vi "Stop all movement.vi"(8 "error in (no error)":errorcluster, 11 "Scientifica XYZ Gen1 in":refnum<class "Scientifica XYZ Gen1.lvclass">) -> (0 "error out":errorcluster, 2 "XYZ Position Set":T1={"Speed"=0, "Z Limit (um+/-)"=0.0, "Axes"="All", "XYZ Coordinates"={"X"=0.0, "Y"=0.0, "Z"=0.0}} {"XYZ Coordinates"."Z" format="Z= %#_g"; "XYZ Coordinates"."Y" format="Y= %#_g"; "XYZ Coordinates"."X" format="X= %#_g"; "Z Limit (um+/-)" format="Z Limit = %.0f"; "Speed" format="Speed= %.0f"}, 3 "Scientifica XYZ Gen1 out":refnum<class "Scientifica XYZ Gen1.lvclass">)   [LabVIEW 2020, in "TranslationStageClassStructure.lvlib" / "Scientifica XYZ Gen1.lvclass"]
uses:
  Scientifica XYZ Gen1.lvclass
  XYZ Stage Control/typedefs/XYZ_position_input.ctl
  XYZ Stage Control/typedefs/XYZ axes.ctl
  Typedefs/XYZ_coordinates.ctl
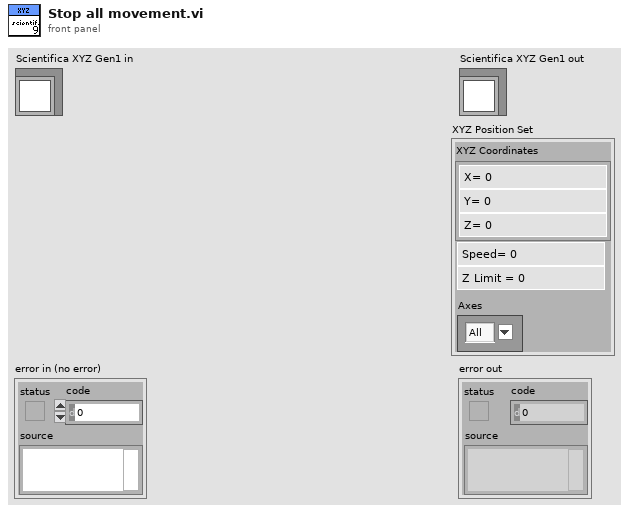
[diagram p1: front panel]
types:
  T1 = typedef "XYZ_position_input.ctl" = cluster{"Speed":i32, "Z Limit (um+/-)":sgl, "Axes":T2, "XYZ Coordinates":T3}
  T2 = typedef "XYZ axes.ctl" = string
  T3 = typedef "XYZ_coordinates.ctl" = cluster{"X":sgl, "Y":sgl, "Z":sgl}
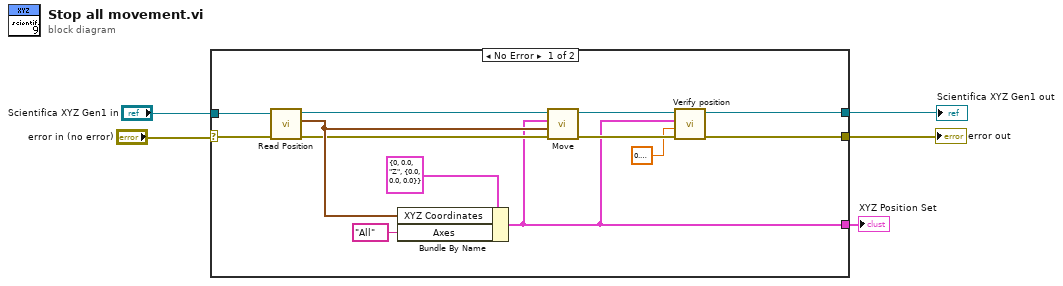
[diagram p0: block diagram]
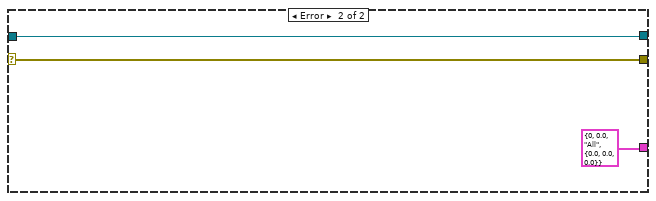
[diagram p2: hidden frame]
diagram:
  n1 = case shown="No Error" "error in (no error)" {
    selector: "error in (no error)" -> [w17 w21]
    tunnel: [w7 w21] -> w4
    tunnel: "Scientifica XYZ Gen1 in" -> [w18 w20]
    tunnel: [w9 w20] -> w2
    tunnel: [w6 T1 {"Speed"=0, "Z Limit (um+/-)"=0.0, "Axes"="All", "XYZ Coordinates"={"X"=0.0, "Y"=0.0, "Z"=0.0}} ("XYZ Position Input")] -> w1
    frame No Error {
      n2 = call-dynamic "Read Position.vi"("error in (no error)"=w17, "Scientifica XYZ Gen1 in"=w18) -> ("error out"=w12:errorcluster, "XYZ Coordinates"=w13:T3, "Scientifica XYZ Gen1 out"=w16:refnum<class "Scientifica XYZ Gen1.lvclass">)  [unwired: 6 in, 1 out]
      n3 = Bundle By Name(cluster=T1 {"Speed"=0, "Z Limit (um+/-)"=0.0, "Axes"="Z", "XYZ Coordinates"={"X"=0.0, "Y"=0.0, "Z"=0.0}} ("XYZ Position Input"), "XYZ Coordinates"=w13, "Axes"=T2 "All") -> (w6:T1)
      n4 = call-dynamic "Move.vi"("error in (no error)"=w12, "Current XYZ Position"=w13, "XYZ Position Input"=w6, "Scientifica XYZ Gen1 in"=w16) -> ("error out"=w11:errorcluster, "Scientifica XYZ Gen1 out"=w10:refnum<class "Scientifica XYZ Gen1.lvclass">)  [unwired: 5 in, 1 out]
      n5 = call-dynamic "Verify position.vi"("error in (no error)"=w11, "Tolerance (um)"=sgl 0.4, "XYZ Position Input"=w6, "Scientifica XYZ Gen1 in"=w10) -> ("error out"=w7:errorcluster, "Scientifica XYZ Gen1 out"=w9:refnum<class "Scientifica XYZ Gen1.lvclass">)  [unwired: 4 in, 2 out]
    }
    frame Error {
    }
  }
  "error out" <- w4
  "Scientifica XYZ Gen1 out" <- w2
  "XYZ Position Set" <- w1
